vi "ArthOps.vi"() -> ()   [LabVIEW 2025]
panel:
  out "floor(x): largest int <= x":dbl
  out "x-1":dbl
  out "x*2^n":dbl
  in  "x":dbl
  in  "y":dbl
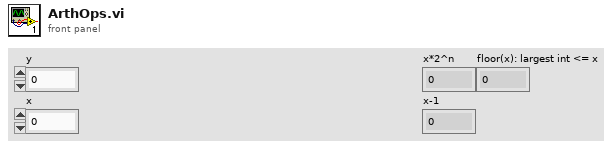
[diagram p1: front panel]
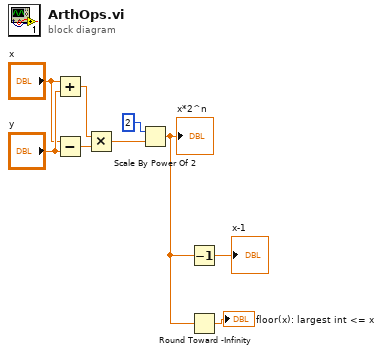
[diagram p0: block diagram]
diagram:
  n1 = Add(x="x", y="y") -> (x+y=w7:dbl)
  n2 = Subtract(x="x", y="y") -> (x-y=w6:dbl)
  n3 = Multiply(x=w7, y=w6) -> (x*y=w5:dbl)
  n4 = Scale By Power Of 2(n=i16 2, x=w5) -> (x*2^n=w2:dbl)
  "x*2^n" <- w2
  n5 = Decrement(x=w2) -> (x-1=→"x-1":dbl)
  n6 = Round Toward -Infinity(1:w2) -> (0:→"floor(x): largest int <= x":dbl)
